vi "NAVX.vi"(10 "navx states":T1) -> (2 "Yaw":dbl)   [LabVIEW 2017]
uses:
  navx states.ctl
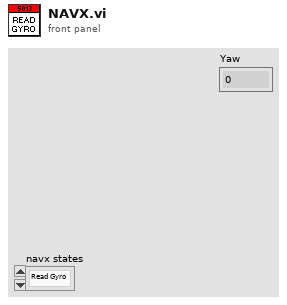
[diagram p1: front panel]
types:
  T1 = typedef "navx states.ctl" = enum16{"Read Gyro", "Reset Gyro"}
  T2 = cluster{"Yaw":dbl, "Roll":dbl, "Pitch":dbl, "Heading":dbl, "Fused Heading":dbl}
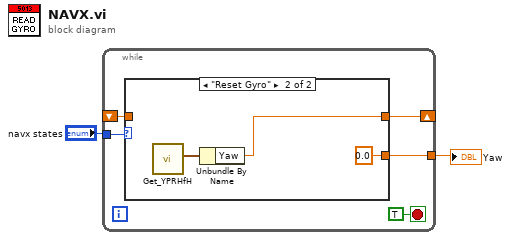
[diagram p0: block diagram]
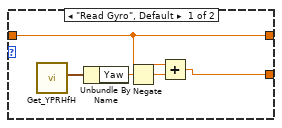
[diagram p2: hidden frame]
diagram:
  n1 = while {
    shift-right: [w4] -> _
    shift-left: _ -> [w3]
    tunnel: "navx states" -> [w6]
    tunnel: [w5] -> w1
    stop <- TRUE stop-if-true
    n2 = case shown="\"Reset Gyro\"" w6 {
      tunnel: [w10 0.0 ("Yaw")] -> w5
      tunnel: [w9 w13] -> w4
      tunnel: w3 -> [w9 _]
      frame "Read Gyro", Default {
        n3 = call <vilib>:"Get_YPRHfH.vi"() -> ("YRPHfH"=w12:T2)  [unwired: 11 in]
        n4 = Unbundle By Name(w12) -> ("Yaw"=w11:dbl)
        n5 = Negate(x=w11) -> (-x=w8:dbl)
        n6 = Add(x=w9, y=w8) -> (x+y=w10:dbl)
      }
      frame "Reset Gyro" {
        n7 = call <vilib>:"Get_YPRHfH.vi"() -> ("YRPHfH"=w15:T2)  [unwired: 11 in]
        n8 = Unbundle By Name(w15) -> ("Yaw"=w13:dbl)
      }
    }
  }
  "Yaw" <- w1
